vi "Removed Serial server.vi"() -> ()   [LabVIEW 2013]
doc: "This is the FPGA VI for the 10-Tap 8-Bit Camera with DRAM example. This example demonstrates how to acquire images from a 10-tap, 8-bit, extended configuration, Camera Link camera and transfer the images to the host. This example supports area scan and line scan cameras for both continuous and finite acquisitions.\n\nThis example also demonstrates the use of DRAM as a frame buffer for very high speed acquisitions. Data packing and flow-control are also employed to maximize use of the available DRAM and FIFOs in terms of both memory space and performance.\n\nAdditionally, the example demonstrates the serial server, which allows third-party camera configuration utilities to communicate with the camera using the Camera Link serial interface while this VI is running."
uses:
  Common/CL Signal Mapping.ctl
  Common/CL Configuration.ctl
  FPGA/Sector/Accumulate/Sector Parameter Cluster.ctl
  <vilib>/Platform/TimedLoop/XDataNode/timing_clust.ctl
  <vilib>/Platform/TimedLoop/XDataNode/nitl_modes.ctl
  <vilib>/Platform/TimedLoop/XDataNode/wakeup.ctl
  FPGA/10-Tap Data/10-Tap Conversion Enum.ctl
  <vilib>/rvi/Emulation/niFpgaSctlEmulationGetInTimedLoop.vi
  <vilib>/rvi/Emulation/niFpgaEmulationReportErrorSimple.vi
  <vilib>/rvi/Emulation/niFpgaGetClockAttributes.vi
  <vilib>/rvi/Emulation/niFpgaCriticalErrorInLSC.vi
  <vilib>/rvi/eio/common/nirviEmuTemplateMethod_errors.vi
  <vilib>/rvi/interface/RandomDataEmulation/nirviRandomDataFPGAFIFO.vi
  <vilib>/rvi/interface/RandomDataEmulation/niFpgaRandomDataHandleErrors.vi
  Common/CL Data to Pixels/10 Tap 8-Bit.vi
  <vilib>/rvi/FIFO/Fifo_Resource/nirvififoEmulationWriteFpgaImpl.vi
  <vilib>/rvi/DataTransferAndStorage/Container/Common/niFpgaContainerGetUniqueNameForEmu.vi
  <vilib>/rvi/FIFO/Fifo_Resource/nirvififoEmulationGetNumberOfElementsToReadFpgaImpl.vi
  <vilib>/rvi/FIFO/Fifo_Resource/nirvififoEmulationReadFpgaImpl.vi
  <vilib>/rvi/FIFO/Fifo_Resource/nirvififoEmulationGetNumberOfElementsToWriteFpgaImpl.vi
  FPGA/Globals/Wing Square Wave Frequency Global.vi
  <vilib>/rvi/Emulation/niFpgaProcessEmulError.vi
  FPGA/Globals/Sector Parameter Global.vi
  FPGA/Globals/Accumulated Sector Intensity.vi
  FPGA/Globals/Pixel Location Global.vi
  <vilib>/Platform/TimedLoop/XDataNode/XDataNode.xnode
  <vilib>/eio/EIONode/EIONode.xnode
  <vilib>/rvi/DataTransferAndStorage/Container/XNode/niFpgaContainer.xnode
  <vilib>/rvi/interface/RandomDataEmulation/nirviRandomDataFpgaReadWriteTemplate.vi
  <vilib>/rvi/FIFO/Fifo_Resource/nirvififoEmulationWrite.vi
  <vilib>/rvi/FIFO/Fifo_Resource/nirvififoEmulationGetNumberOfElementsToRead.vi
  <vilib>/rvi/FIFO/Fifo_Resource/nirvififoEmulationRead.vi
  <vilib>/rvi/FIFO/Fifo_Resource/nirvififoEmulationGetNumberOfElementsToWrite.vi
  <vilib>/Platform/TimedLoop/XDataNode/XDNodeRunTimeDep.lvlib
panel:
  in  "[Average BG Intensity]":u8[](array[numeric])=[0, 0, 0, 0, 0, 0, 0, 0, 0, 0, 0, 0, 0, 0, 0, 0, 0, 0, 0, 0, 0, 0, 0, 0, 0, 0, 0, 0, 0, 0, 0, 0]
  in  "Sector Threshold":u8
  in  "# of Frames to Average":u8
  in  "Sector Parameters Right":T1={"Start Angle"=0.13543701171875, "End Angle"=0.30462646484375, "Inner Radius"=309, "Outter Radius"=405, "Hinge X"=1106, "Hinge Y"=803, "NumWingSectors"=8}
  in  "Sector Parameters Left":T1={"Start Angle"=0.6541748046875, "End Angle"=0.856201171875, "Inner Radius"=309, "Outter Radius"=405, "Hinge X"=947, "Hinge Y"=829, "NumWingSectors"=8}
  in  "Sim":bool=TRUE
  in  "CL Config.Configuration":T2=enum."Full"
  in  "CL Config.Signal Mapping":T3=enum."Basler 10-tap"
  in  "CL Config.Line Scan":bool
  in  "CL Config.DVAL Active High":bool=TRUE
  in  "CL Config.LVAL Active High":bool=TRUE
  in  "CL Config.FVAL Active High":bool=TRUE
  in  "CL Config.Spare Active High":bool=TRUE
  in  "Acq Control.Line Scan Height":u32
  in  "Acq Control.Frames To Acq":u32
  in  "Acq Control.Acquire":bool
  in  "Acq Control.Cancel Acq":bool
  in  "Acq Control.Ignore DVAL":bool
  in  "Acq Control.Initialize":bool
  out "Acq Status.Acq In Progress":bool
  out "Acq Status.Clocks Per Line":u32
  out "Acq Status.Frames Acq'd":u32
  out "Acq Status.Lines Per Frame":u32
  out "Acq Status.DMA Write Timeout":bool
  out "Acq Status.Initialized":bool
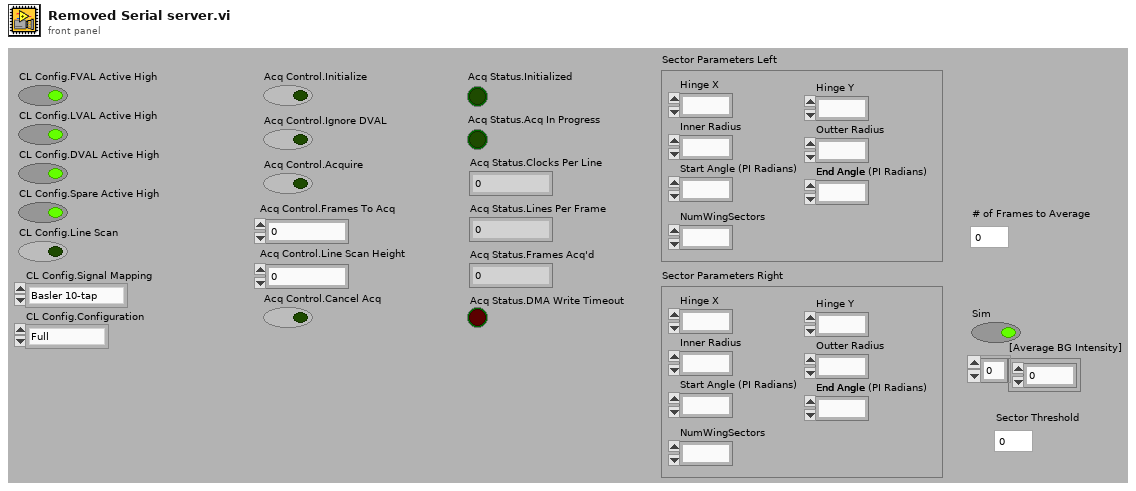
[diagram p1: front panel]
types:
  T1 = typedef "Sector Parameter Cluster.ctl" = cluster{"Start Angle":fxp<+,17,3>, "End Angle":fxp<+,17,3>, "Inner Radius":u16, "Outter Radius":u16, "Hinge X":u16, "Hinge Y":u16, "NumWingSectors":u8}
  T2 = typedef "CL Configuration.ctl" = enum8{"Base", "Medium", "Full"}
  T3 = typedef "CL Signal Mapping.ctl" = enum8{"Standard", "Basler 10-tap", "Vosskühler 10-tap"}
  T4 = typedef "XDNodeRunTimeDep.lvlib/timing_clust.ctl" = cluster{"Expected End [f-1]":u64, "Actual End [f-1]":u64, "Finished Late? [f-1]":bool, "Expected End [i-1]":u64, "Actual End [i-1]":u64, "Finished Late? [i-1]":bool, "Expected Start [i]":u64, "Actual Start [i]":u64, "Expected Start [f]":u64, "Actual Start [f]":u64, "Source Name":string, "Structure Name":string, "Period":i64, "Deadline":i64, "Offset":i64, "Start":i64, "Priority":i32, "Timeout":i32, "Mode":T5, "Wakeup Reason":T6, "Error":errorcluster, "Source Type":string, "Secondary Source Type":string, "Global End Time":u64, "Global Start Time":u64, "Frame Duration":u64, "Iteration Duration":u64, "Assigned CPU":i32, "I/O Scan Engine Mode":u32}
  T5 = typedef "XDNodeRunTimeDep.lvlib/nitl_modes.ctl" = enum32{"No Change", "Process missed periods, maintain original phase", "Discard missed periods, maintain original phase", "Process missed periods, ignore original phase", "Discard missed periods, ignore original phase"}
  T6 = typedef "XDNodeRunTimeDep.lvlib/wakeup.ctl" = enum32{"Normal", "Aborted", "Asynchronous wakeup", "Timing source error", "Timed loop error", "Timeout"}
  T7 = typedef "10-Tap Conversion Enum.ctl" = enum16{"10-Tap to 16 and 64", "16 and 64 to 10-Tap"}
  T8 = cluster{"Enables Valid":bool, "Frame Valid":bool, "Line Valid":bool, "Data Valid":bool}
  T9 = typedef "10-Tap 8-bit Cluster.ctl" = cluster{"Pixel 0":u8, "Pixel 1":u8, "Pixel 2":u8, "Pixel 3":u8, "Pixel 4":u8, "Pixel 5":u8, "Pixel 6":u8, "Pixel 7":u8, "Pixel 8":u8, "Pixel 9":u8}
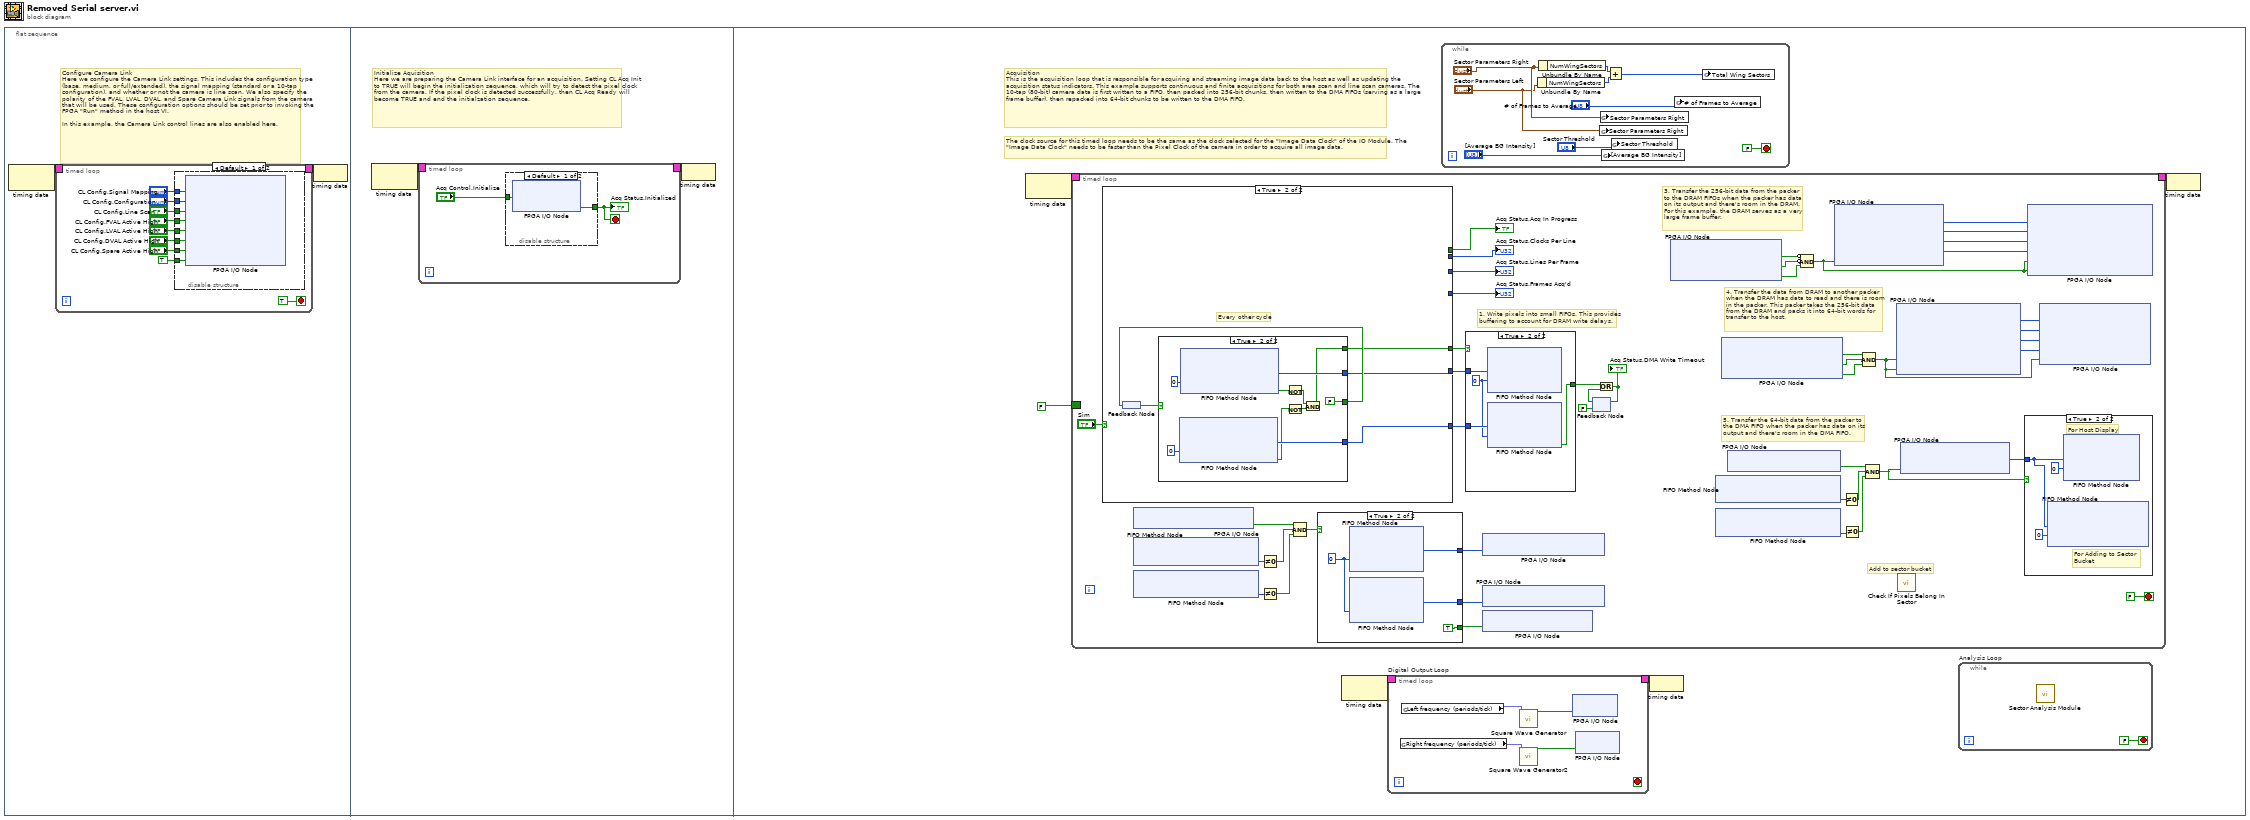
[diagram p0: block diagram]
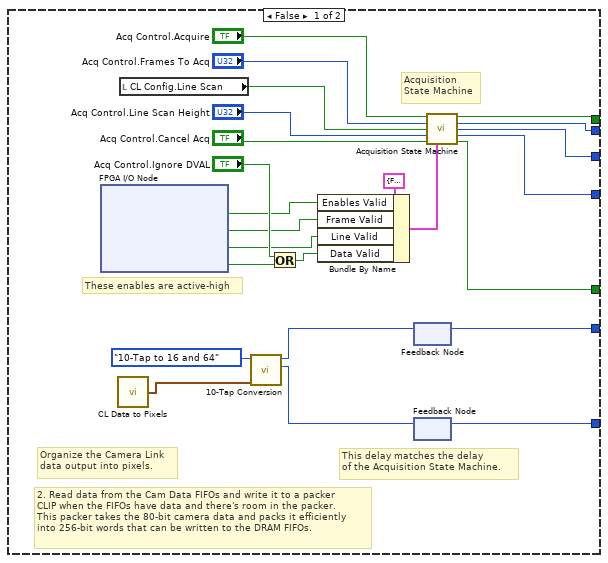
[diagram p5: hidden frame]
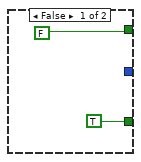
[diagram p6: hidden frame]
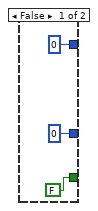
[diagram p7: hidden frame]
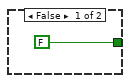
[diagram p8: hidden frame]
diagram:
  n1 = flat-sequence {
    frame #0 {
      # "Configure Camera Link\nHere we configure the Camera Link settings. This includes the configuration type (base, medium, or full/extended), the signal mapping (standard or a 10-tap configuration), and whether or not the camera is line scan. We also specify the polarity of the FVAL, LVAL, DVAL, and Spare Camera Link signals from the camera that will be used. These configuration options should be set prior to invoking the FPGA \"Run\" method in the host VI.\n\nIn this example, the Camera Link control lines are also enabled here."
      n2 = node-c288() -> (w2:T4)  [unwired: 1 in]
      n3 = timed-loop {
        timing: w2 -> [_]
        timing-out: [_] -> w1
        stop <- TRUE stop-if-true
        n4 = disable-structure shown="Default" {
          disable-tunnel: "CL Config.FVAL Active High" -> [w19 _]
          disable-tunnel: "CL Config.LVAL Active High" -> [w18 _]
          disable-tunnel: "CL Config.DVAL Active High" -> [w17 _]
          disable-tunnel: "CL Config.Spare Active High" -> [w16 _]
          disable-tunnel: "CL Config.Signal Mapping" -> [w15 _]
          disable-tunnel: "CL Config.Configuration" -> [w14 _]
          disable-tunnel: "CL Config.Line Scan" -> [w13 _]
          disable-tunnel: TRUE ("IO Module\\CL Control Enable") -> [w12 _]
          frame condition #0 (active) {
            n5 = xnode "FPGA I/O Node"("CL Set Signal Mapping"=w15, "CL Set Configuration"=w14, "CL Set Line Scan"=w13, "CL Set FVAL Active High"=w19, "CL Set LVAL Active High"=w18, "CL Set DVAL Active High"=w17, "CL Set Spare Active High"=w16, "CL Control Enable"=w12) -> ()  [unwired: 8 in, 8 out]
          }
          frame condition #1 {
          }
        }
      }
      n6 = node-c288(w1) -> ()
    }
    frame #1 {
      # "Initialize Aquisition\nHere we are preparing the Camera Link interface for an acquisition. Setting CL Acq Init to TRUE will begin the initialization sequence, which will try to detect the pixel clock from the camera. If the pixel clock is detected successfully, then CL Acq Ready will become TRUE and end the initialzation sequence."
      n7 = node-c288() -> (w25:T4)  [unwired: 1 out]
      n8 = timed-loop {
        timing: w25 -> [_]
        timing-out: [_] -> w24
        stop <- w26 stop-if-true
        n9 = disable-structure shown="Default" {
          disable-tunnel: "Acq Control.Initialize" -> [w29 w30]
          disable-tunnel: [w28 w30] -> w26
          frame condition #0 (active) {
            n10 = xnode "FPGA I/O Node"("CL Acq Init"=w29) -> ("CL Acq Ready"=w28:bool)  [unwired: 2 in, 2 out]
          }
          frame condition #1 {
          }
        }
        "Acq Status.Initialized" <- w26
      }
      n11 = node-c288(w24) -> ()
    }
    frame #2 {
      # "The clock source for this timed loop needs to be the same as the clock selected for the \"Image Data Clock\" of the IO Module. The \"Image Data Clock\" needs to be faster than the Pixel Clock of the camera in order to acquire all image data."
      # "Acquisition\nThis is the acquisition loop that is responsible for acquiring and streaming image data back to the host as well as updating the acquisition status indicators. This example supports continuous and finite acquisitions for both area scan and line scan cameras. The 10-tap (80-bit) camera data is first written to a FIFO, then packed into 256-bit chunks, then written to the DMA FIFOs (serving as a large frame buffer), then repacked into 64-bit chunks to be written to the DMA FIFO."
      n12 = node-c288() -> (w39:T4)  [unwired: 1 in]
      n13 = timed-loop {
        timing: w39 -> [_]
        timing-out: [_] -> w38
        border: FALSE -> [_]
        stop <- FALSE stop-if-true
        # "Add to sector bucket"
        # "5. Transfer the 64-bit data from the packer to\nthe DMA FIFO when the packer has data on its\noutput and there's room in the DMA FIFO."
        # "4. Transfer the data from DRAM to another packer\nwhen the DRAM has data to read and there is room\nin the packer. This packer takes the 256-bit data\nfrom the DRAM and packs it into 64-bit words for\ntransfer to the host."
        # "3. Transfer the 256-bit data from the packer\nto the DRAM FIFOs when the packer has data\non its output and there's room in the DRAM.\nFor this example, the DRAM serves as a very\nlarge frame buffer."
        # "1. Write pixels into small FIFOs. This provides\nbuffering to account for DRAM write delays."
        n14 = case shown="True" "Sim" {
          tunnel: [w128 w129] -> w101
          tunnel: [w127 w130] -> w96
          tunnel: [w109 w132] -> w84
          tunnel: [w113 _] -> w83
          tunnel: [w112 _] -> w82
          tunnel: [w111 _] -> w81
          tunnel: [w110 _] -> w80
          frame False {
            # "These enables are active-high"
            # "Acquisition\nState Machine"
            # "2. Read data from the Cam Data FIFOs and write it to a packer\nCLIP when the FIFOs have data and there's room in the packer.\nThis packer takes the 80-bit camera data and packs it efficiently\ninto 256-bit words that can be written to the DRAM FIFOs."
            # "Organize the Camera Link\ndata output into pixels."
            # "This delay matches the delay\nof the Acquisition State Machine."
            n15 = xnode "FPGA I/O Node"() -> ("CL Output Valid"=w117:bool, "CL Frame Valid"=w118:bool, "CL Line Valid"=w119:bool, "CL Data Valid"=w122:bool)  [unwired: 4 in, 4 out]
            n16 = call-poly "CL Data to Pixels.vi"() -> ("Pixels"=w105:T9)  [unwired: 1 in]
            n17 = local read "CL Config.Line Scan"() -> (w125:bool)
            n18 = call "10-Tap Conversion.vi"("10 Tap In"=w105, "Operation"=10-Tap_Conversion_Enum."10-Tap to 16 and 64") -> ("64 Bit Out"=w106:u64, "16 Bit Out"=w107:u16)  [unwired: 7 in, 1 out]
            n19 = Or(x="Acq Control.Ignore DVAL", y=w122) -> (x .or. y?=w123:bool)
            n20 = Bundle By Name(cluster=T8 {"Enables Valid"=FALSE, "Frame Valid"=FALSE, "Line Valid"=FALSE, "Data Valid"=FALSE} ("Enables"), "Enables Valid"=w117, "Frame Valid"=w118, "Line Valid"=w119, "Data Valid"=w123) -> (w120:T8)
            n21 = feedback #1() -> (w127:u16)  [unwired: 1 in]
            n22 = feedback-in #1(w107) -> ()
            n23 = feedback #2() -> (w128:u64)  [unwired: 1 in]
            n24 = feedback-in #2(w106) -> ()
            n25 = call "Acquisition State Machine.vi"("Acquire"="Acq Control.Acquire", "Frames to Acquire"="Acq Control.Frames To Acq", "Line Scan"=w125, "Line Scan Height"="Acq Control.Line Scan Height", "Cancel Acq"="Acq Control.Cancel Acq", "Enables"=w120) -> ("Acq In Progress"=w113:bool, "Num Clocks Per Line"=w112:u32, "Num Lines Per Frame"=w111:u32, "Num Frames Acq'd"=w110:u32, "Capture Cycle"=w109:bool)  [unwired: 4 in, 1 out]
          }
          frame True {
            # "Every other cycle"
            n26 = feedback #3() -> (w131:bool)
            n27 = case shown="True" w131 {
              tunnel: [_ w145] -> w130
              tunnel: [_ w144] -> w129
              tunnel: [FALSE w137] -> w132
              tunnel: [TRUE FALSE] -> w133
              frame False {
              }
              frame True {
                n28 = xnode ("FIFO Method Node")("Timeout"=0) -> ("Element"=w144:u64, "Timed Out?"=w140:bool)  [unwired: 1 in, 1 out]
                n29 = xnode ("FIFO Method Node")("Timeout"=0) -> ("Element"=w145:u16, "Timed Out?"=w141:bool)  [unwired: 1 in, 1 out]
                n30 = Not(x=w141) -> (.not. x?=w139:bool)
                n31 = Not(x=w140) -> (.not. x?=w138:bool)
                n32 = And(x=w139, y=w138) -> (x .and. y?=w137:bool)
              }
            }
            n33 = feedback-in #3(w133) -> ()
          }
        }
        "Acq Status.Frames Acq'd" <- w80
        "Acq Status.Lines Per Frame" <- w81
        "Acq Status.Clocks Per Line" <- w82
        "Acq Status.Acq In Progress" <- w83
        n34 = xnode "FPGA I/O Node"() -> ("Pack 80 to 256\\Ready For Write"=w90:bool)  [unwired: 1 in, 1 out]
        n35 = xnode ("FIFO Method Node")() -> ("Number of Elements to Read"=w94:u32)  [unwired: 1 in, 1 out]
        n36 = xnode ("FIFO Method Node")() -> ("Number of Elements to Read"=w93:u32)  [unwired: 1 in, 1 out]
        n37 = Not Equal To 0?(x=w94) -> (x != 0?=w88:bool)
        n38 = Not Equal To 0?(x=w93) -> (x != 0?=w87:bool)
        n39 = Compound Arithmetic op=AND(w90, w88, w87) -> (w89:bool)
        n40 = case shown="True" w89 {
          tunnel: [u16 0 ("Element") w152] -> w95
          tunnel: [u64 0 ("Element") w151] -> w91
          tunnel: [FALSE TRUE] -> w92
          frame False {
          }
          frame True {
            w150 = 0 ("Timeout")
            n41 = xnode ("FIFO Method Node")("Timeout"=w150) -> ("Element"=w152:u16)  [unwired: 1 in, 2 out]
            n42 = xnode ("FIFO Method Node")("Timeout"=w150) -> ("Element"=w151:u64)  [unwired: 1 in, 2 out]
          }
        }
        n43 = case shown="True" w84 {
          tunnel: [FALSE ("Timed Out?") w156] -> w99
          tunnel: w101 -> [_ w157]
          tunnel: w96 -> [_ w155]
          frame False {
          }
          frame True {
            w154 = 0 ("Timeout")
            n44 = xnode ("FIFO Method Node")("Element"=w155, "Timeout"=w154) -> ()  [unwired: 1 in, 2 out]
            n45 = xnode ("FIFO Method Node")("Element"=w157, "Timeout"=w154) -> ("Timed Out?"=w156:bool)  [unwired: 1 in, 1 out]
          }
        }
        n46 = xnode "FPGA I/O Node"("Pack 80 to 256\\Data In Upper 16"=w95) -> ()  [unwired: 1 in, 1 out]
        n47 = xnode "FPGA I/O Node"("Pack 80 to 256\\Data In Lower 64"=w91) -> ()  [unwired: 1 in, 1 out]
        n48 = xnode "FPGA I/O Node"("Pack 80 to 256\\Write Enable"=w92) -> ()  [unwired: 1 in, 1 out]
        n49 = feedback #4(FALSE) -> (w98:bool)
        n50 = Or(x=w99, y=w98) -> (x .or. y?=w97:bool)
        "Acq Status.DMA Write Timeout" <- w97
        n51 = feedback-in #4(w97) -> ()
        n52 = xnode "FPGA I/O Node"() -> ("DRAM Bank 0\\Full"=w60:bool, "Pack 80 to 256\\Output Valid"=w79:bool)  [unwired: 3 in, 4 out]
        n53 = xnode ("FIFO Method Node")() -> ("Number of Elements to Write"=w62:u32)  [unwired: 1 in, 1 out]
        n54 = xnode ("FIFO Method Node")() -> ("Number of Elements to Write"=w59:u32)  [unwired: 1 in, 1 out]
        n55 = xnode "FPGA I/O Node"() -> ("DRAM Bank 1\\Data_Available"=w73:bool, "DRAM Bank 0\\Data_Available"=w71:bool, "Pack 256 To 64\\Ready for Write"=w72:bool)  [unwired: 3 in, 3 out]
        n56 = xnode "FPGA I/O Node"() -> ("Pack 256 To 64\\Output Valid"=w64:bool)  [unwired: 1 in, 1 out]
        n57 = Compound Arithmetic op=AND(invert w60, invert w60, w79) -> (w74:bool)
        n58 = xnode "FPGA I/O Node"("Pack 80 to 256\\Read Enable"=w74) -> ("Pack 80 To 256\\Data Out 3"=w78:u64, "Pack 80 To 256\\Data Out 2"=w77:u64, "Pack 80 To 256\\Data Out 1"=w76:u64, "Pack 80 To 256\\Data Out 0"=w75:u64)  [unwired: 5 in, 5 out]
        n59 = Not Equal To 0?(x=w62) -> (x != 0?=w63:bool)
        n60 = Not Equal To 0?(x=w59) -> (x != 0?=w58:bool)
        n61 = Compound Arithmetic op=AND(w73, w71, w72) -> (w66:bool)
        n62 = Compound Arithmetic op=AND(w64, w63, w58) -> (w61:bool)
        n63 = xnode "FPGA I/O Node"("DRAM Bank 1\\Read"=w66, "DRAM Bank 0\\Read"=w66) -> ("DRAM Bank 1\\Read_Data_Upper"=w70:u64, "DRAM Bank 1\\Read_Data_Lower"=w69:u64, "DRAM Bank 0\\Read_Data_Upper"=w68:u64, "DRAM Bank 0\\Read_Data_Lower"=w67:u64)  [unwired: 6 in, 6 out]
        n64 = call "Check If Pixels Belong In Sector.vi"() -> ()  [unwired: 11 in, 1 out]
        n65 = xnode "FPGA I/O Node"("Pack 256 to 64\\Read Enable"=w61) -> ("Pack 256 To 64\\Data Out 64"=w65:u64)  [unwired: 2 in, 2 out]
        n66 = case shown="True" w61 {
          tunnel: w65 -> [_ w103]
          frame False {
          }
          frame True {
            # "For Adding to Sector \nBucket"
            # "For Host Display"
            n67 = xnode ("FIFO Method Node")("Element"=w103, "Timeout"=0) -> ()  [unwired: 1 in, 2 out]
            n68 = xnode ("FIFO Method Node")("Element"=w103, "Timeout"=0) -> ()  [unwired: 1 in, 2 out]
          }
        }
        n69 = xnode "FPGA I/O Node"("DRAM Bank 1\\Write_Data_Upper"=w78, "DRAM Bank 1\\Write_Data_Lower"=w77, "DRAM Bank 0\\Write_Data_Upper"=w76, "DRAM Bank 0\\Write_Data_Lower"=w75, "DRAM Bank 1\\Write"=w74, "DRAM Bank 0\\Write"=w74) -> ()  [unwired: 6 in, 6 out]
        n70 = xnode "FPGA I/O Node"("Pack 256 To 64\\Data In 3"=w70, "Pack 256 To 64\\Data In 2"=w69, "Pack 256 To 64\\Data In 1"=w68, "Pack 256 To 64\\Data In 0"=w67, "Pack 256 to 64\\Write Enable"=w66) -> ()  [unwired: 5 in, 5 out]
      }
      n71 = node-c288() -> (w36:T4)  [unwired: 1 in]
      n72 = timed-loop "Digital Output Loop" {
        timing: w36 -> [_]
        timing-out: [_] -> w35
        stop <- _ stop-if-true
        n73 = global read "Wing Square Wave Frequency Global.vi" "Right frequency (periods/tick)"() -> (w50:fxp<+,32,0>)
        n74 = global read "Wing Square Wave Frequency Global.vi" "Left frequency (periods/tick)"() -> (w51:fxp<+,32,0>)
        n75 = call "Square Wave Generator"("frequency (periods/tick)"=w51) -> ("square wave out"=w53:bool)  [unwired: 14 in]
        n76 = call "Square Wave Generator2"("frequency (periods/tick)"=w50) -> ("square wave out"=w52:bool)  [unwired: 14 in]
        n77 = xnode "FPGA I/O Node"("TTL 0"=w53) -> ()  [unwired: 1 in, 1 out]
        n78 = xnode "FPGA I/O Node"("TTL 1"=w52) -> ()  [unwired: 1 in, 1 out]
      }
      n79 = while {
        stop <- FALSE stop-if-true
        n80 = Unbundle By Name("Sector Parameters Left") -> ("NumWingSectors"=w46:u8)
        n81 = Unbundle By Name("Sector Parameters Right") -> ("NumWingSectors"=w47:u8)
        n82 = global write "Sector Parameter Global.vi" "Sector Parameters Right"("Sector Parameters Left") -> ()
        n83 = global write "Sector Parameter Global.vi" "Sector Parameters Right"("Sector Parameters Right") -> ()
        n84 = global write "Sector Parameter Global.vi" "[Average BG Intensity]"("[Average BG Intensity]") -> ()
        n85 = Add(x=w47, y=w46) -> (x+y=w45:u8)
        n86 = global write "Sector Parameter Global.vi" "Sector Threshold"("Sector Threshold") -> ()
        n87 = global write "Pixel Location Global.vi" "# of Frames to Average"("# of Frames to Average") -> ()
        n88 = global write "Accumulated Sector Intensity.vi" "Total Wing Sectors"(w45) -> ()
      }
      n89 = node-c288(w35) -> ()
      n90 = while "Analysis Loop" {
        stop <- FALSE stop-if-true
        n91 = call "Sector Analysis Module.vi"() -> ()  [unwired: 11 in, 1 out]
      }
      n92 = node-c288(w38) -> ()
    }
  }
